vi "WriteNearFar.vi"(1 "本次文件名":string) -> ()   [LabVIEW 2018]
uses:
  Init/AllPath.vi
  Reslut.vi
  <vilib>/Utility/file.llb/Write Delimited Spreadsheet (string).vi
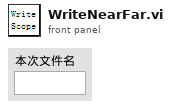
[diagram p1: front panel]
types:
  T1 = typedef "IMAQ Image.ctl" = refnum<image>
  T2 = cluster{"近场图":T1, " 远场图":T1, "发散角X/rad":dbl, "发散角Y/rad":dbl}
  T3 = cluster{"能量/功率":path, " 示波器":path, " 光谱仪":path, "偏振":path, "近远场":cluster{" 近场图片":path, " 远场图片":path, "发散角数据":path}, "参数":path, " 基路径":path, "文件名信息":path}
  T4 = cluster{"激光器型号":string, "X":dbl, "Y":dbl, "Z":dbl, "Rotate":dbl, "Pitching":dbl}
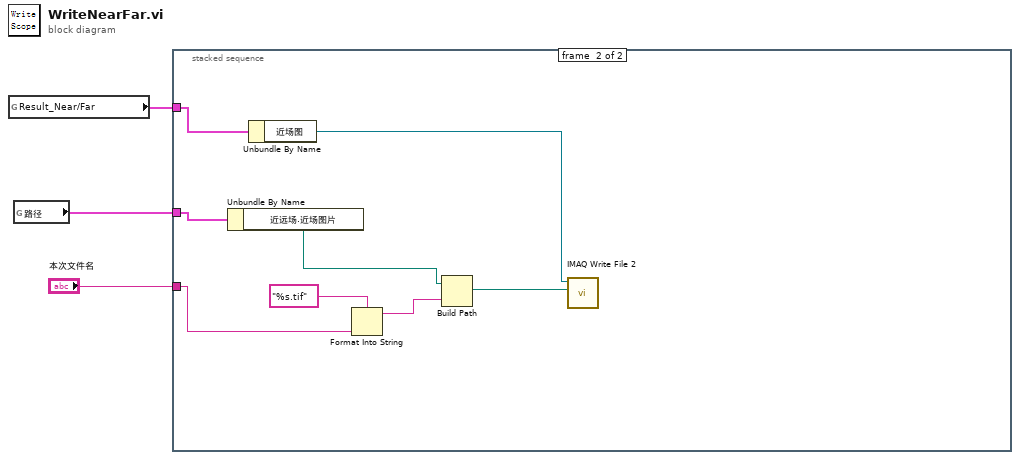
[diagram p0: block diagram]
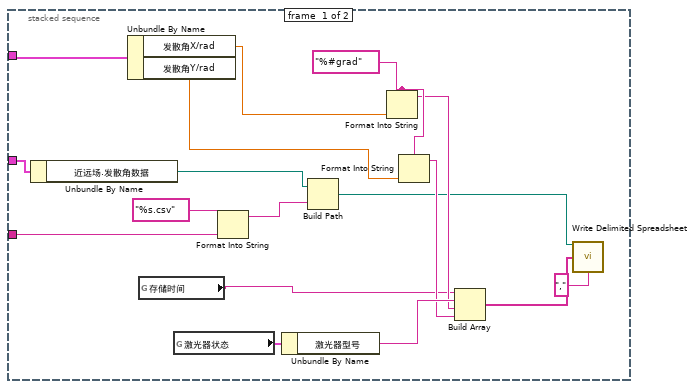
[diagram p2: hidden frame]
diagram:
  n1 = global read "Reslut.vi" "Result_Near/Far"() -> (w2:T2)
  n2 = global read "AllPath.vi" "路径"() -> (w3:T3)
  n3 = stacked-sequence {
    tunnel: w3 -> [w20 w28]
    tunnel: w2 -> [w17 w27]
    tunnel: "本次文件名" -> [w15 w23]
    frame #0 {
      w11 = "%#grad" ("格式字符串")
      n4 = Unbundle By Name(w20) -> ("近远场.发散角数据"=w19:path)
      n5 = Unbundle By Name(w17) -> ("发散角X/rad"=w12:dbl, "发散角Y/rad"=w10:dbl)
      n6 = global read "Reslut.vi" "存储时间"() -> (w4:string)
      n7 = global read "参数.vi" "激光器状态"() -> (w18:T4)
      n8 = Format Into String(format string="%s.csv" ("格式字符串"), w15) -> (resulting string=w14:string)  [unwired: 2 in, 1 out]
      n9 = Unbundle By Name(w18) -> ("激光器型号"=w13:string)
      n10 = Build Path(base path=w19, name or relative path=w14) -> (appended path=w7:path)
      n11 = Format Into String(format string=w11, w12) -> (resulting string=w9:string)  [unwired: 2 in, 1 out]
      n12 = Format Into String(format string=w11, w10) -> (resulting string=w8:string)  [unwired: 2 in, 1 out]
      n13 = Build Array(w4, w13, w9, w8) -> (w6:string[])
      n14 = call-poly <vilib>:"Write Delimited Spreadsheet.vi"("file path (dialog if empty)"=w7, "1D data"=w6, "delimiter (\\t)"="," ("delimiter (\\t)")) -> ()  [unwired: 11 in, 2 out]
    }
    frame #1 {
      n15 = Unbundle By Name(w28) -> ("近远场.近场图片"=w25:path)
      n16 = Unbundle By Name(w27) -> ("近场图"=w22:T1)
      n17 = Format Into String(format string="%s.tif" ("格式字符串"), w23) -> (resulting string=w26:string)  [unwired: 2 in, 1 out]
      n18 = Build Path(base path=w25, name or relative path=w26) -> (appended path=w21:path)
      n19 = call-poly "IMAQ Write File 2"("File Path"=w21, "Image"=w22) -> ()  [unwired: 8 in, 2 out]
    }
  }
